vi "Property of node_2_0.vi"() -> ()   [LabVIEW 2015]
panel:
  in  "stop":bool
  in  "Tab Control":enum32{"Page 1", "Page 2"}(tab)
  in  "String":string
  out "String 2":string
  out "length":i32
  in  "Visible":bool
  # "Length of string with Property of Node-2"
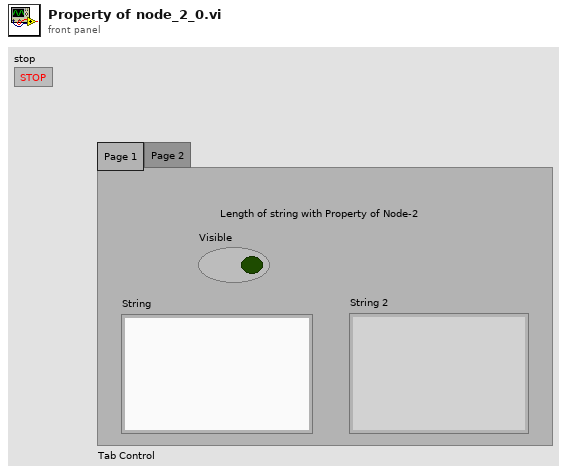
[diagram p1: front panel]
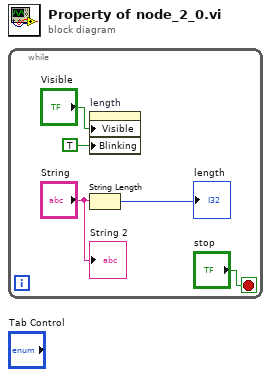
[diagram p0: block diagram]
diagram:
  n1 = while {
    stop <- "stop" stop-if-true
    n2 = property on="length" class="DigNum (strict)"("Visible"="Visible", "Blinking"=TRUE) -> ()  [unwired: 2 in, 2 out]
    n3 = String Length(string="String") -> (length=→"length":i32)
    "String 2" <- "String"
  }
